vi "UsrProfiles-Import profile dialogue 26_01_18.vi"(8 "error in (no error)":errorcluster) -> (0 "error out":errorcluster, 1 "cancelled":bool, 2 "target filepath":path, 3 "Source filepath":path caption="selected path")   [LabVIEW 2017]
uses:
  <userlib>/_MGI/File/MGI Windows Folder Enum.ctl
  Typedefs/Which path.ctl
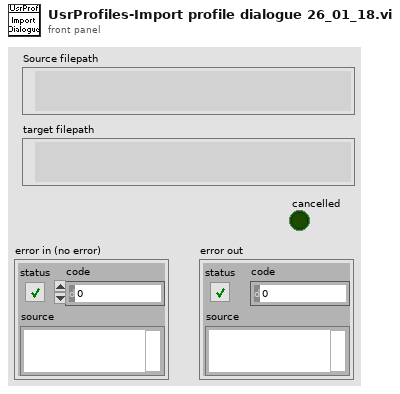
[diagram p1: front panel]
types:
  T1 = typedef "MGI Windows Folder Enum.ctl" = enum32{"Desktop", "Err<Internet>", "Programs", "Err<Controls>", "Err<Printers>", "Personal (MyDocuments)", "Favorites", "Startup", "Recent", "SendTo", "Err<RecycleBin>", "StartMenu", "Err<MyDocuments>", "MyMusic", "MyVideo", "Err<0x000F>", "DesktopDirectory", "Err<Drives>", "Err<Network>", "NetHood", "Fonts", "Templates", "CommonStartMenu", "CommonPrograms", "CommonStartup", "CommonDesktopDirectory", "AppData", "PrintHood", "LocalAppData", "Err<AltStartup>", "Err<CommonAltStartup>", "CommonFavorites", "InternetCache", "Cookies", "History", "CommonAppData", "Windows", "System", "ProgramFiles", "MyPictures", "Profile", "System32", "Err<0x002A>", "ProgramFilesCommon", "Err<0x002C>", "CommonTemplates", "CommonDocuments", "CommonAdminTools", "AdminTools"}
  T2 = typedef "Which path.ctl" = enum16{"Configuration Files", "Calibration Files", "Images", "Setup.ini", "Loaded User profile.ini", "User's-Previous session.ini", "New user profile.ini", "Selected User profile.ini", "User profiles folder", "Power meter scaling.txt", "FOV Cal.ini", "Calibration.ini"}
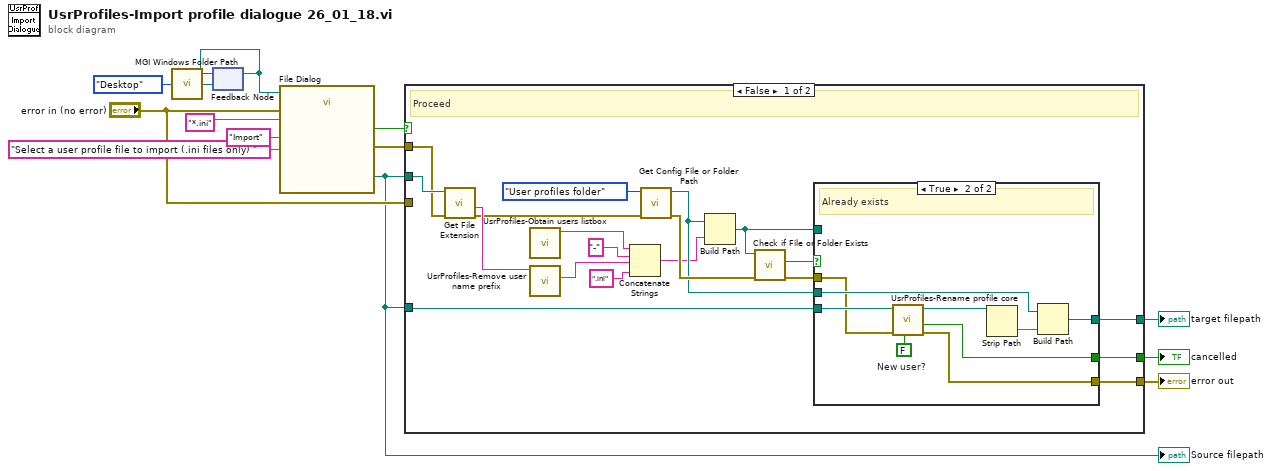
[diagram p0: block diagram]
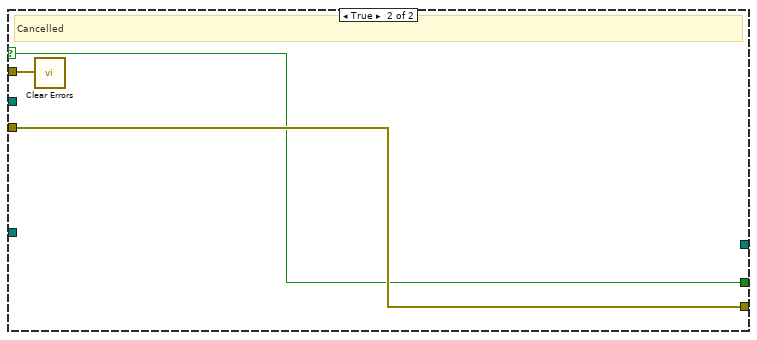
[diagram p3: hidden frame]
diagram:
  n1 = call <userlib>:"MGI Windows Folder Path.vi"("Windows Folder"=MGI_Windows_Folder_Enum."Desktop") -> ("Path"=w6:path)
  n2 = feedback #1(w6) -> (w5:path)
  n3 = feedback-in #1(w5) -> ()
  n4 = call "File Dialog"("start path"=w5, "prompt"="Select a user profile file to import (.ini files only) ", "button label"="Import", "error in"="error in (no error)", "pattern (all files)"="*.ini" ("pattern label")) -> ("selected path"=w2:path, "cancelled"=w7:bool, "error out"=w9:errorcluster)  [unwired: 7 in, 1 out]
  "Source filepath" <- w2
  n5 = case shown="False" w7 {
    selector: w7 -> [_ w44]
    tunnel: w2 -> [w22 _]
    tunnel: [w27 _] -> w10
    tunnel: w9 -> [w20 w46]
    tunnel: [w14 w45] -> w8
    tunnel: "error in (no error)" -> [_ w45]
    tunnel: w2 -> [w29 _]
    tunnel: [w25 w44] -> w1
    frame False {
      # "Proceed"
      n6 = call <vilib>:"Get File Extension.vi"("error in (no error)"=w20, "file"=w22) -> ("error out"=w19:errorcluster, "filename without extension"=w21:string)  [unwired: 5 in, 3 out]
      n7 = call "UsrProfiles-Obtain users listbox.vi"() -> ("Selected user's name"=w16:string)  [unwired: 8 in, 3 out]
      n8 = call "UsrProfiles-Remove user name prefix.vi"("Profile name (full)"=w21) -> ("Profile name (user removed)"=w18:string)  [unwired: 10 in]
      n9 = Concatenate Strings(w16, "-" ("string"), w18, ".ini" ("string")) -> (w24:string)
      n10 = call "Get Config File or Folder Path.vi"("Error In"=w19, "Which file or folder?"=Which_path."User profiles folder" ("Which file?")) -> ("Error Out"=w30:errorcluster, "File Path"=w28:path)  [unwired: 7 in, 1 out]
      n11 = Build Path(base path=w28, name or relative path=w24) -> (appended path=w26:path)
      n12 = call <vilib>:"Check if File or Folder Exists.vi"("error in (no error)"=w30, "path"=w26) -> ("error out"=w15:errorcluster, "file or folder exists?"=w31:bool)  [unwired: 7 in, 1 out]
      n13 = case shown="True" w31 {
        tunnel: w29 -> [_ w42]
        tunnel: w28 -> [_ w39]
        tunnel: [w34 w38] -> w27
        tunnel: w26 -> [w34 _]
        tunnel: [_ w37] -> w25
        tunnel: w15 -> [w33 w36]
        tunnel: [w33 w35] -> w14
        frame False {
          # "OK to import"
        }
        frame True {
          w43 = FALSE  # New user?
          # "Already exists"
          n14 = call "UsrProfiles-Rename profile core.vi"("New user"=w43, "error in (no error)"=w36, "Source profile's filepath"=w42) -> ("error out"=w35:errorcluster, "Cancelled"=w37:bool, "Filepath of profile to be created"=w41:path)  [unwired: 5 in, 1 out]
          n15 = Strip Path(path=w41) -> (name=w40:string)  [unwired: 1 out]
          n16 = Build Path(base path=w39, name or relative path=w40) -> (appended path=w38:path)
        }
      }
    }
    frame True {
      # "Cancelled"
      n17 = call <vilib>:"Clear Errors.vi"("error in (no error)"=w46) -> ()  [unwired: 5 in, 2 out]
    }
  }
  "error out" <- w8
  "target filepath" <- w10
  "cancelled" <- w1
